vi "_PC_Spectrafilter enable_draw_rectangle.vi"(8 "error in (no error)":errorcluster, 9 "mouse type":enum16{"none", "down", "move", "up"}(ring), 10 "Coords":T1, 11 "xy graph ref":refnum<vi>) -> (0 "error out":errorcluster, 1 "max value":dbl, 2 "min value":dbl)   [LabVIEW 2018]
uses:
  <vilib>/Utility/miscctls.llb/LVPoint32TypeDef.ctl
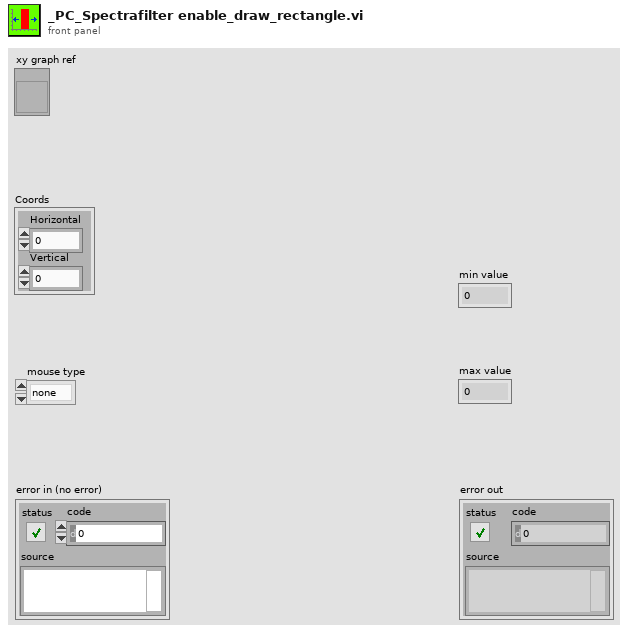
[diagram p1: front panel]
types:
  T1 = typedef "LVPoint32TypeDef.ctl" = cluster{"Horizontal":i32, "Vertical":i32}
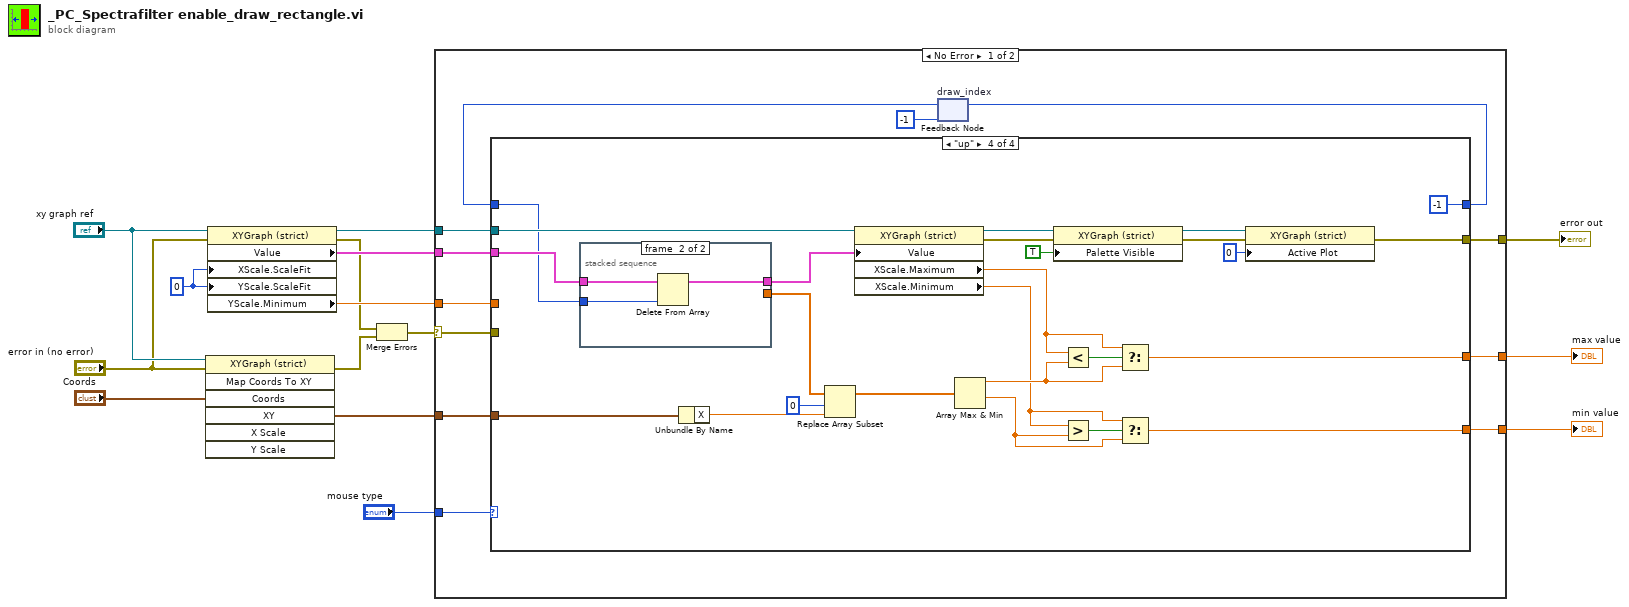
[diagram p0: block diagram]
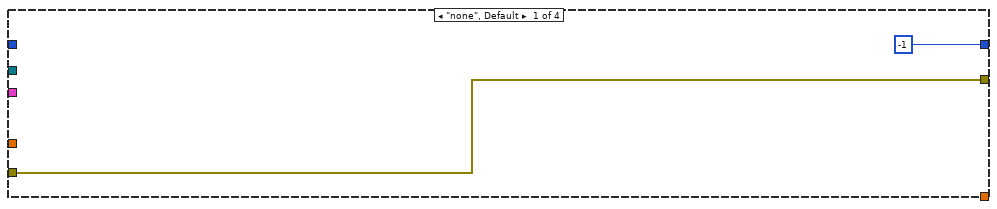
[diagram p2: hidden frame]
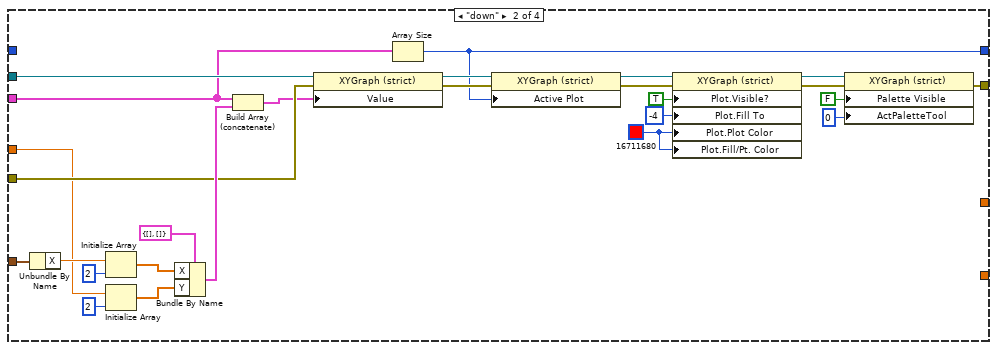
[diagram p3: hidden frame]
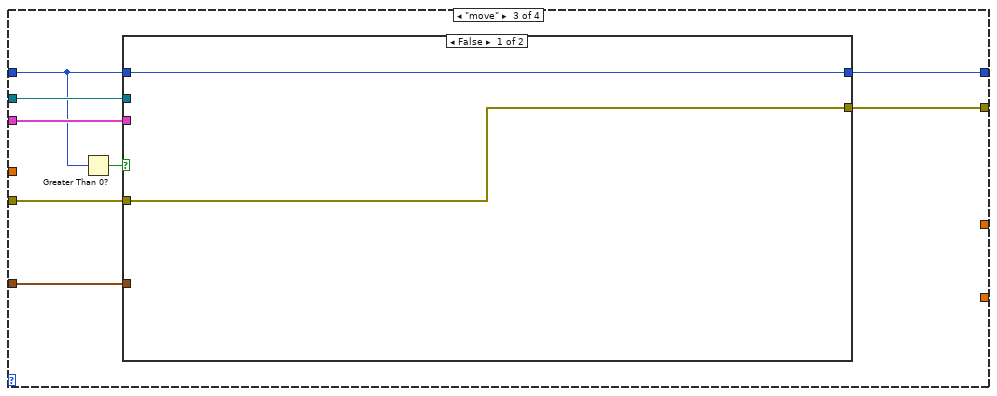
[diagram p4: hidden frame]
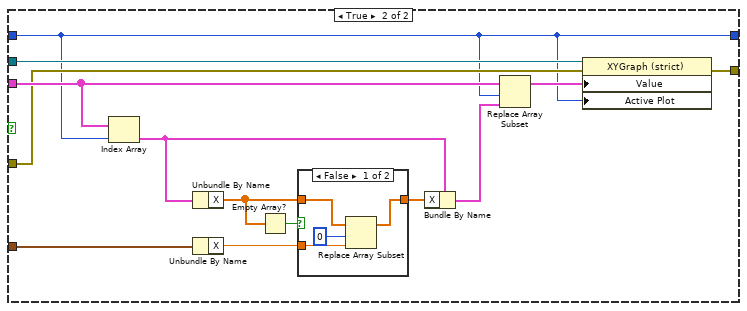
[diagram p5: hidden frame]
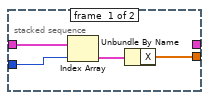
[diagram p7: hidden frame]
diagram:
  w13 = u8 0 ("X Scale.Scale Fit")
  n1 = invoke class="XYGraph (strict)" method="Map Coords To XY"(reference="xy graph ref", error in="error in (no error)", "Coords"="Coords") -> (error out=w5:errorcluster, "XY"=w7:cluster{"X":dbl, "Y":dbl})  [unwired: 4 in, 5 out]
  n2 = property class="XYGraph (strict)"(reference="xy graph ref", error in="error in (no error)", "XScale.ScaleFit"=w13, "YScale.ScaleFit"=w13) -> (reference out=w12:refnum<vi>, error out=w4:errorcluster, "Value"=w10:cluster{"X":dbl[], "Y":sgl[]}[], "YScale.Minimum"=w11:dbl)
  n3 = Merge Errors(w4, w5) -> (w3:errorcluster)
  n4 = case shown="No Error" w3 {
    selector: w3 -> [w19 _]
    tunnel: [w27 _] -> w15
    tunnel: "mouse type" -> [w24 _]
    tunnel: w12 -> [w23 _]
    tunnel: w11 -> [w22 _]
    tunnel: w10 -> [w21 _]
    tunnel: w7 -> [w20 _]
    tunnel: [w18 _] -> w2
    tunnel: [w17 _] -> w1
    frame No Error {
      n5 = feedback #1 "draw_index"(-1) -> (w25:i32)
      n6 = case shown="\"up\"" w24 {
        tunnel: w23 -> [_ w40 w61 w108]
        tunnel: [w29 w43 w59 w84] -> w27
        tunnel: [-1 w31 w56 -1] -> w26
        tunnel: w25 -> [_ _ w57 w91]
        tunnel: w22 -> [_ w38 _ _]
        tunnel: w21 -> [_ w36 w63 w94]
        tunnel: w20 -> [_ w41 w62 w107]
        tunnel: w19 -> [w29 w39 w60 _]
        tunnel: [_ _ _ w97] -> w18
        tunnel: [_ _ _ w96] -> w17
        frame "none", Default {
        }
        frame "down" {
          w30 = u32 16711680
          n7 = Unbundle By Name(w41) -> ("X"=w54:dbl)
          n8 = Initialize Array(w54, 2 ("dimension size")) -> (w50:dbl[])
          n9 = Initialize Array(w38, 2 ("dimension size")) -> (w49:dbl[])
          n10 = Bundle By Name(cluster=cluster{"X":dbl[], "Y":sgl[]} {"X"=[], "Y"=[]} ("new element/subarray"), "X"=w50, "Y"=w49) -> (w42:cluster{"X":dbl[], "Y":sgl[]})
          n11 = Build Array (concatenate)(w36, w42) -> (w37:cluster{"X":dbl[], "Y":sgl[]}[])
          n12 = property class="XYGraph (strict)"(reference=w40, error in=w39, "Value"=w37) -> (reference out=w35:refnum<vi>, error out=w34:errorcluster)
          n13 = Array Size(array=w36) -> (size(s)=w31:i32)
          n14 = property class="XYGraph (strict)"(reference=w35, error in=w34, "Active Plot"=w31) -> (reference out=w33:refnum<vi>, error out=w32:errorcluster)
          n15 = property class="XYGraph (strict)"(reference=w33, error in=w32, "Plot.Visible?"=TRUE ("Visible"), "Plot.Fill To"=i16 -4, "Plot.Plot Color"=w30, "Plot.Fill/Pt. Color"=w30) -> (reference out=w45:refnum<vi>, error out=w44:errorcluster)
          n16 = property class="XYGraph (strict)"(reference=w45, error in=w44, "Palette Visible"=FALSE ("Palette:Visible"), "ActPaletteTool"=0 ("Palette:Active Tool")) -> (error out=w43:errorcluster)  [unwired: 1 out]
        }
        frame "move" {
          n17 = Greater Than 0?(x=w57) -> (x > 0?=w58:bool)
          n18 = case shown="False" w58 {
            tunnel: w63 -> [_ w78]
            tunnel: w62 -> [_ w74]
            tunnel: w61 -> [_ w70]
            tunnel: w60 -> [w64 w69]
            tunnel: [w64 w67] -> w59
            tunnel: w57 -> [w65 w66]
            tunnel: [w65 w66] -> w56
            frame False {
            }
            frame True {
              n19 = Index Array(array=w78, index=w66) -> (element=w72:cluster{"X":dbl[], "Y":sgl[]})
              n20 = Unbundle By Name(w72) -> ("X"=w75:dbl[])
              n21 = Unbundle By Name(w74) -> ("X"=w73:dbl)
              n22 = Empty Array?(array=w75) -> (empty?=w76:bool)
              n23 = case shown="False" w76 {
                tunnel: w73 -> [w81 _]
                tunnel: [w80 w83] -> w77
                tunnel: w75 -> [w79 w83]
                frame False {
                  n24 = Replace Array Subset(array=w79, new element=w81, index=0) -> (w80:dbl[])
                }
                frame True {
                }
              }
              n25 = Bundle By Name(cluster=w72, "X"=w77) -> (w71:cluster{"X":dbl[], "Y":sgl[]})
              n26 = Replace Array Subset(array=w78, new element=w71, index=w66) -> (w68:cluster{"X":dbl[], "Y":sgl[]}[])
              n27 = property class="XYGraph (strict)"(reference=w70, error in=w69, "Value"=w68, "Active Plot"=w66) -> (error out=w67:errorcluster)  [unwired: 1 out]
            }
          }
        }
        frame "up" {
          n28 = stacked-sequence {
            tunnel: w94 -> [w112 w115]
            tunnel: w91 -> [w109 w114]
            tunnel: [_ w113] -> w92
            tunnel: [w110 _] -> w93
            frame #0 {
              n29 = Index Array(array=w112, index=w109) -> (element=w111:cluster{"X":dbl[], "Y":sgl[]})
              n30 = Unbundle By Name(w111) -> ("X"=w110:dbl[])
            }
            frame #1 {
              n31 = Delete From Array(array=w115, index=w114) -> (array with subset deleted=w113:cluster{"X":dbl[], "Y":sgl[]}[])  [unwired: 1 in, 1 out]
            }
          }
          n32 = Unbundle By Name(w107) -> ("X"=w105:dbl)
          n33 = Replace Array Subset(array=w93, new element=w105, index=0) -> (w104:dbl[])
          n34 = property class="XYGraph (strict)"(reference=w108, "Value"=w92) -> (reference out=w90:refnum<vi>, error out=w88:errorcluster, "XScale.Maximum"=w99:dbl, "XScale.Minimum"=w98:dbl)  [unwired: 1 in]
          n35 = Array Max & Min(array=w104) -> (max value=w101:dbl, min value=w100:dbl)  [unwired: 2 out]
          n36 = property class="XYGraph (strict)"(reference=w90, error in=w88, "Palette Visible"=TRUE ("Palette:Visible")) -> (reference out=w87:refnum<vi>, error out=w85:errorcluster)
          n37 = Less?(x=w99, y=w101) -> (x < y?=w103:bool)
          n38 = Greater?(x=w98, y=w100) -> (0:w102:bool)
          n39 = Select(t=w99, s=w103, f=w101) -> (s? t:f=w97:dbl)
          n40 = Select(t=w98, s=w102, f=w100) -> (s? t:f=w96:dbl)
          n41 = property class="XYGraph (strict)"(reference=w87, error in=w85, "Active Plot"=u32 0) -> (error out=w84:errorcluster)  [unwired: 1 out]
        }
      }
      n42 = feedback-in #1(w26) -> ()
    }
    frame Error {
    }
  }
  "error out" <- w15
  "max value" <- w2
  "min value" <- w1
